vi "BuildFastAOtasks.vi"(6 "Input Cluster":T1={"inbits"=8, "outbits"=38, "Counter"="6733_1", "Digital"="6509", "Fast AO"=["6733_1", "6733_2"], "Task Names"=["Inbits", "Outbits", "Counter", "FastAO_1", "FastAO_2"]}, 9 "counter in":tag="/6733_1/PXI_Trig0", 10 "Sample rate":dbl=100000.0, 11 "Task cluster in":T2={"inbits"=8, "outbits"=38, "Counter"="Counter", "Inbits"="Inbits", "Outbits"="Outbits", "Fast AO"=["Fast AO_1", "Fast AO_2"], "Errors"={"status"=FALSE, "code"=0, "source"=""}}) -> (3 "Task cluster out":T2={"inbits"=8, "outbits"=38, "Counter"="Counter", "Inbits"="Inbits", "Outbits"="Outbits", "Fast AO"=["FastAO_1", "FastAO_2"], "Errors"={"status"=FALSE, "code"=0, "source"=""}})   [LabVIEW 2018]
uses:
  Tasks_RT.ctl
  <vilib>/DAQmx/create/channels.llb/DAQmx Create Channel (AO-Voltage-Basic).vi
  <vilib>/DAQmx/configure/timing.llb/DAQmx Timing (Sample Clock).vi
  <resource>/objmgr/daqmx.rc
panel:
  # "Tasks and errors"
  # "Tasks and errors"
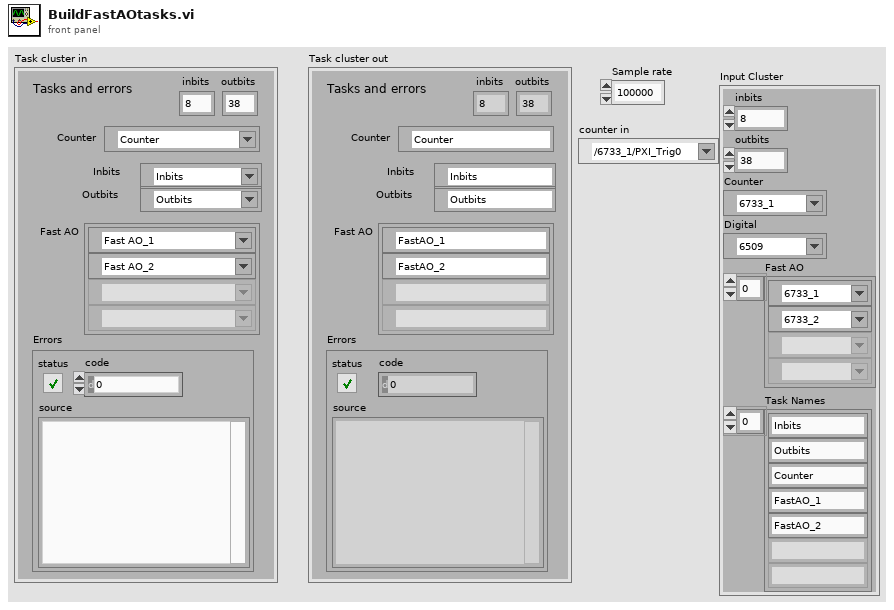
[diagram p1: front panel]
types:
  T1 = cluster{"inbits":i32, "outbits":i32, "Counter":tag, "Digital":tag, "Fast AO":tag[], "Task Names":string[]}
  T2 = typedef "Tasks_RT.ctl" = cluster{"inbits":i32, "outbits":i32, "Counter":refnum<k21>, "Inbits":refnum<k21>, "Outbits":refnum<k21>, "Fast AO":refnum<k21>[], "Errors":errorcluster}
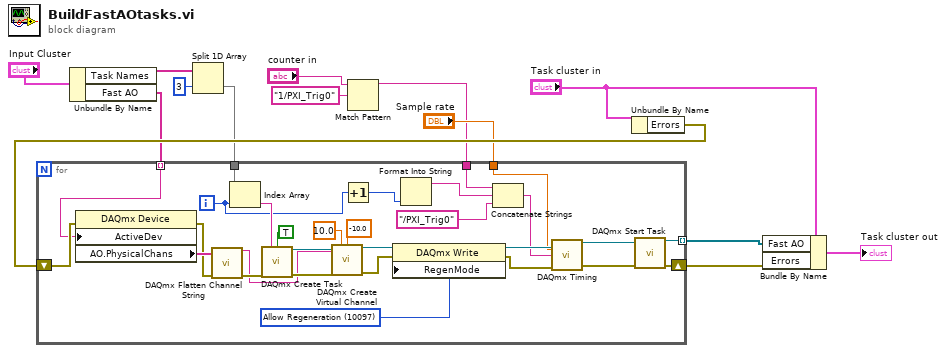
[diagram p0: block diagram]
diagram:
  n1 = Unbundle By Name("Input Cluster") -> ("Task Names"=w8:string[], "Fast AO"=w4:tag[])
  n2 = Split 1D Array(array=w8, index=3) -> (second subarray=w10:string[])  [unwired: 1 out]
  n3 = Match Pattern(string="counter in", regular expression="1/PXI_Trig0") -> (before substring=w1:string)  [unwired: 1 in, 3 out]
  n4 = Unbundle By Name("Task cluster in") -> ("Errors"=w13:errorcluster)
  n5 = for {
    tunnel: w10 -> [w27]
    tunnel: w4 -> [w22] mode=indexing
    tunnel: [w28] -> w11 mode=indexing
    tunnel: "Sample rate" -> [w21]
    shift-right: [w25] -> w14
    shift-left: w13 -> [w23]
    tunnel: w1 -> [w17]
    i -> [w16]
    w43 = 10097 items=["Allow Regeneration"=10097, "Do Not Allow Regeneration"=10158] ("RegenMode")
    n6 = property class="DAQmx Device"(error in=w23, "ActiveDev"=w22) -> (error out=w30:errorcluster, "AO.PhysicalChans"=w31:tag[])  [unwired: 1 in, 1 out]
    n7 = call <vilib>:"DAQmx Flatten Channel String.vi"("names in"=w31, "error in"=w30) -> ("names out"=w29:string, "error out"=w40:errorcluster)  [unwired: 12 in]
    n8 = Index Array(array=w27, index=w16) -> (element=w26:string)
    n9 = call <vilib>:"DAQmx Create Task.vi"("new task name"=w26, "auto cleanup"=TRUE, "error in"=w40) -> ("task out"=w38:refnum<k21>, "error out"=w39:errorcluster)  [unwired: 11 in]
    n10 = call-poly <vilib>:"DAQmx Create Virtual Channel.vi"("task in"=w38, "maximum value"=10.0, "minimum value"=-10.0, "physical channels"=w29, "error in"=w39) -> ("task out"=w36:refnum<k21>, "error out"=w35:errorcluster)  [unwired: 9 in]
    n11 = Increment(x=w16) -> (x+1=w20:i32)
    n12 = property class="DAQmx Write"(reference=w36, error in=w35, "RegenMode"=w43) -> (reference out=w34:refnum<k21>, error out=w33:errorcluster)
    n13 = Format Into String(w20) -> (resulting string=w18:string)  [unwired: 3 in, 1 out]
    n14 = Concatenate Strings(w17, w18, "/PXI_Trig0" ("regular expression")) -> (w15:string)
    n15 = call-poly <vilib>:"DAQmx Timing.vi"("task/channels in"=w34, "rate"=w21, "source"=w15, "error in"=w33) -> ("task out"=w24:refnum<k21>, "error out"=w32:errorcluster)  [unwired: 10 in]
    n16 = call <vilib>:"DAQmx Start Task.vi"("task/channels in"=w24, "error in"=w32) -> ("task out"=w28:refnum<k21>, "error out"=w25:errorcluster)  [unwired: 12 in]
  }
  n17 = Bundle By Name(cluster="Task cluster in", "Fast AO"=w11, "Errors"=w14) -> (→"Task cluster out":T2)
